vi "test Endpoint_Connected_Sends Connected Message.vi"(8 "error in (no error)":errorcluster, 11 "TestCase in":refnum<class "Test Legacy Nested Endpoint.lvclass">) -> (0 "error out":errorcluster, 3 "TestCase out":refnum<class "Test Legacy Nested Endpoint.lvclass">)   [LabVIEW 2020, in "Test Legacy Nested Endpoint.lvclass"]
uses:
  Test Legacy Nested Endpoint.lvclass
  <vilib>/addons/_JKI Toolkits/VI Tester/TestCase.llb/TestCase.lvclass
  <vilib>/ActorFramework/Message Queue/Message Queue.lvclass
  <vilib>/ActorFramework/Message Dequeuer/Message Dequeuer.lvclass
  Source/Legacy Nested Endpoint/Legacy Nested Endpoint Messages/Connected Msg/Connected Msg.lvclass
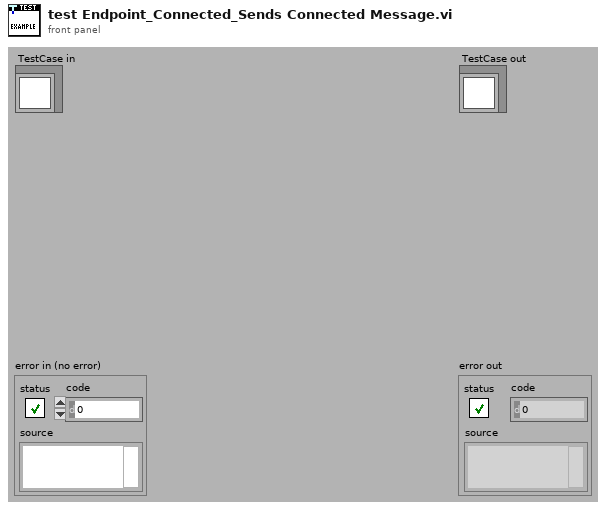
[diagram p1: front panel]
types:
  T1 = cluster{"Endpoint Enqueuer":refnum<class "Message Enqueuer.lvclass">}
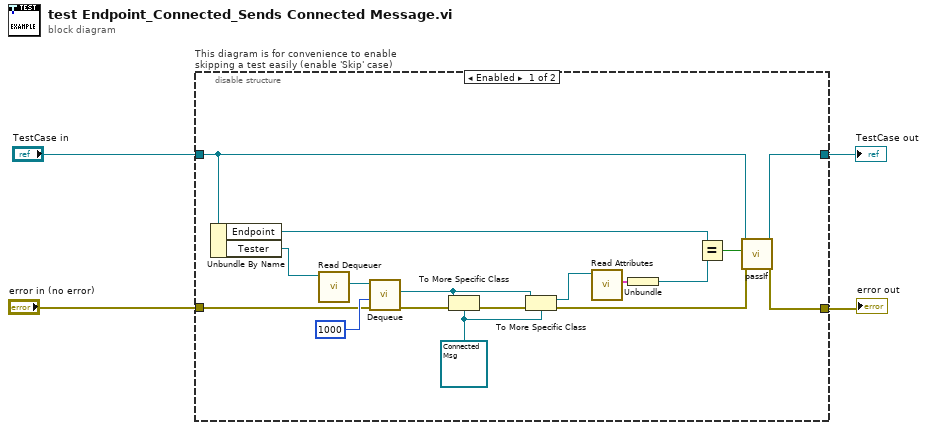
[diagram p0: block diagram]
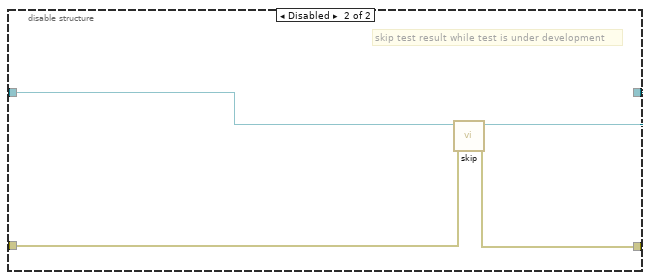
[diagram p2: hidden frame]
diagram:
  n1 = disable-structure "This diagram is for convenience to enable skipping a test easily (enable 'Skip' case)" shown="Enabled" {
    disable-tunnel: "TestCase in" -> [w19 w25]
    disable-tunnel: [w21 w23] -> w1
    disable-tunnel: [w20 w24] -> w3
    disable-tunnel: "error in (no error)" -> [w8 w22]
    frame Enabled {
      w11 = refnum<class "Connected Msg.lvclass"> refnum ("Nested Endpoint.lvlib:Connected Msg.lvclass")
      n2 = Unbundle By Name(w19) -> ("Endpoint"=w5:refnum<class "Message Enqueuer.lvclass">, "Tester"=w18:refnum<class "Message Queue.lvclass">)
      n3 = call <vilib>:"Read Dequeuer.vi"("Message Queue"=w18) -> ("Message Dequeuer"=w17:refnum<class "Message Dequeuer.lvclass">)  [unwired: 10 in]
      n4 = call <vilib>:"Dequeue.vi"("error in (no error)"=w8, "timeout in ms (-1)"=1000, "Message Dequeuer in"=w17) -> ("error out"=w14:errorcluster, "Message"=w12:refnum<class "Message.lvclass">)  [unwired: 4 in, 3 out]
      n5 = To More Specific Class(target class=w11, reference=w12, error in=w14) -> (error out=w13:errorcluster)  [unwired: 1 out]
      n6 = To More Specific Class(target class=w11, reference=w12, error in=w13) -> (specific class reference=w10:refnum<class "Connected Msg.lvclass">, error out=w7:errorcluster)
      n7 = call "Read Attributes.vi"("Connected Msg"=w10) -> ("Payload"=w9:T1)  [unwired: 10 in]
      n8 = Unbundle(w9) -> ("Endpoint Enqueuer"=w6:refnum<class "Message Enqueuer.lvclass">)
      n9 = Equal?(x=w5, y=w6) -> (x = y?=w16:bool)
      n10 = call-dynamic "passIf.vi"("error in (no error)"=w7, "pass"=w16, "TestCase in"=w19) -> ("error out"=w20:errorcluster, "TestCase out"=w21:refnum<class "Test Legacy Nested Endpoint.lvclass">)  [unwired: 7 in]
    }
    frame Disabled {
      # "skip test result while test is under development"
      n11 = call <vilib>:"skip.vi"("error in (no error)"=w22, "TestCase in"=w25) -> ("error out"=w24:errorcluster, "TestCase out"=w23:refnum<class "Test Legacy Nested Endpoint.lvclass">)  [unwired: 8 in]
    }
  }
  "error out" <- w3
  "TestCase out" <- w1
